vi "[FGV] Control_Eanble_Disable.vi"(7 "Control_EnDisable_Action":T2, 8 "Error In":errorcluster, 10 "Tab":T1=enum."Lookup Table", 11 "This VI":refnum<vi>) -> (0 "Error Out":errorcluster, 3 "PageRefOut":refnum<vi>)   [LabVIEW 2019]
uses:
  Controls/Control_EnDisable_Action.ctl
  Controls/UI_Process_Type.ctl
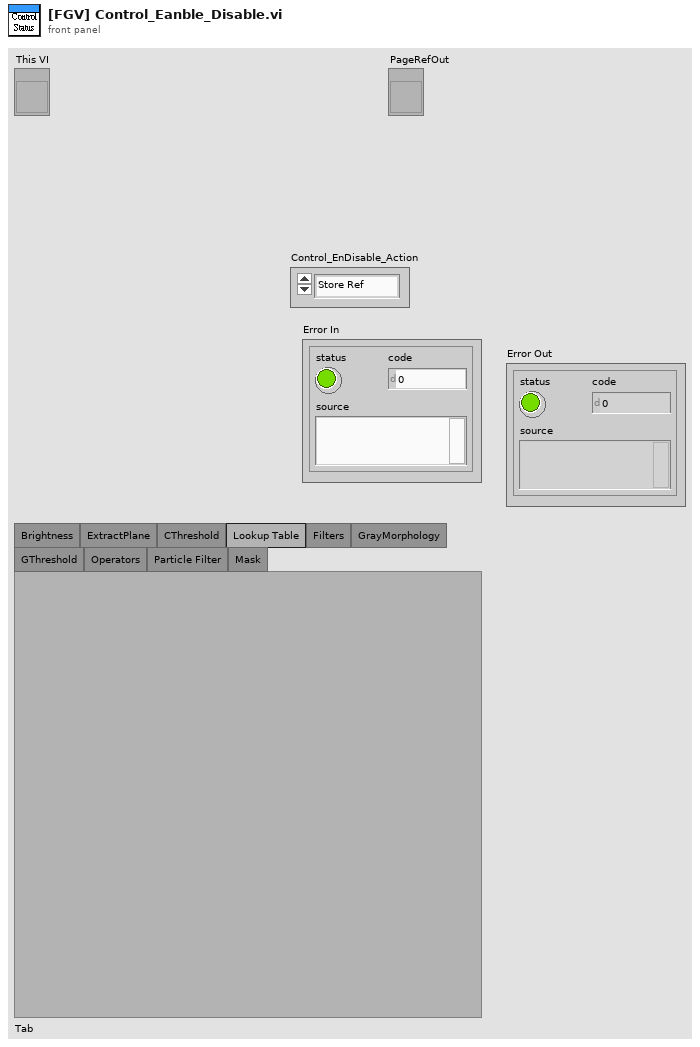
[diagram p1: front panel]
types:
  T1 = typedef "UI_Process_Type.ctl" = enum32{"None", "Brightness", "ExtractPlane", "CThreshold", "Lookup Table", "Filters", "GrayMorphology", "GThreshold", "Operators", "Particle Filter", "Mask"}
  T2 = typedef "Control_EnDisable_Action.ctl" = enum16{"Store Ref", "Add Mode", "Select Mode", "Enable All", "OnePageEnable", "OnePageDisable", "AllPageDisable", "AllPageEnable", "PageRefOut"}
  T3 = enum8{"Enabled", "Disabled", "Disabled and Grayed Out"}
  T4 = enum32{"Page Enabled", "Page Disabled", "Page Disabled & Grayed"}
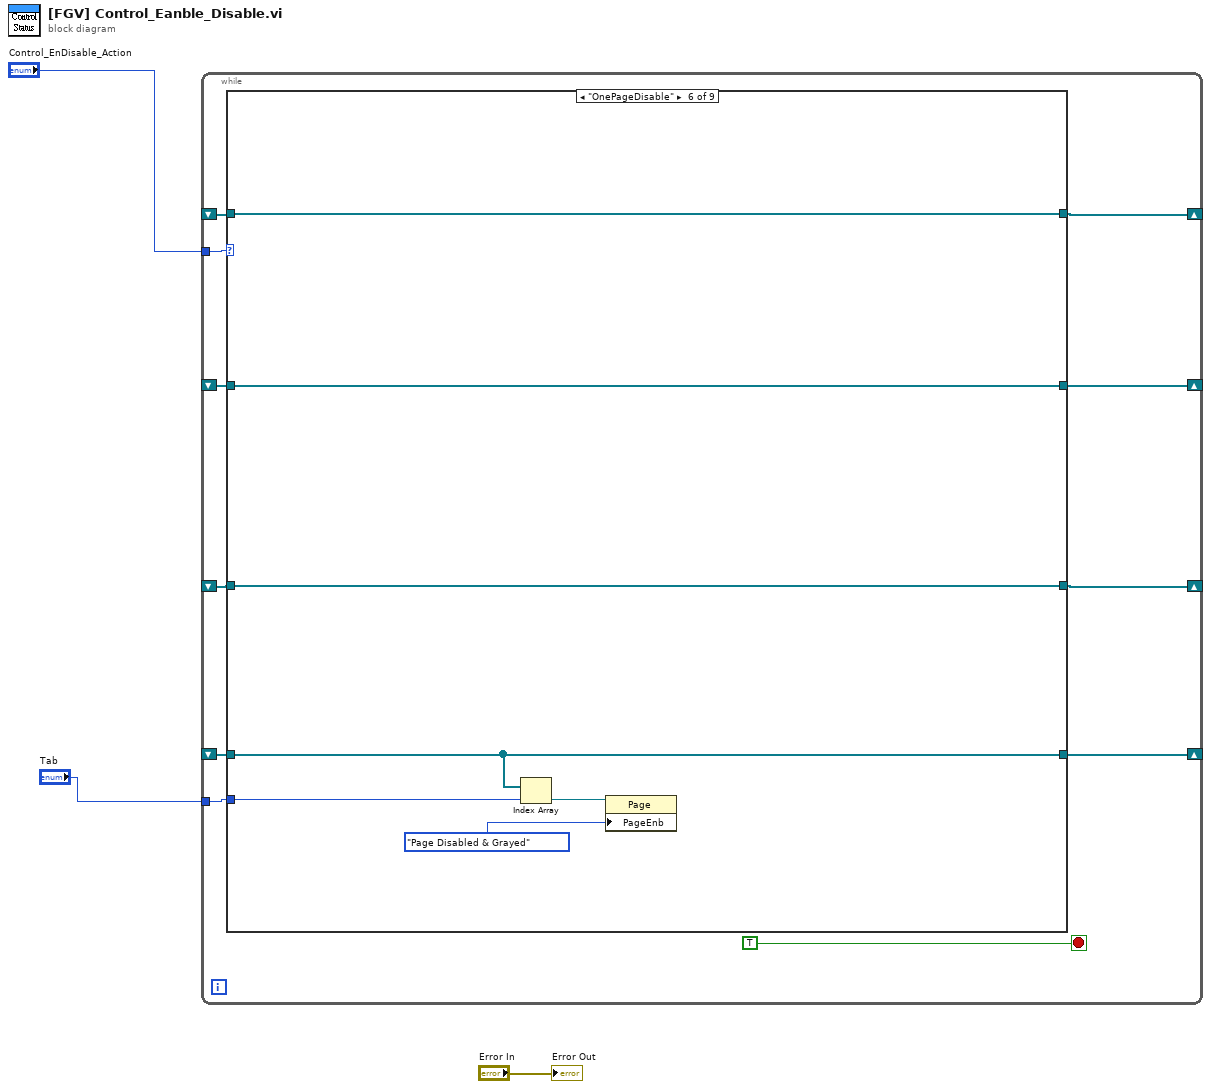
[diagram p0: block diagram]
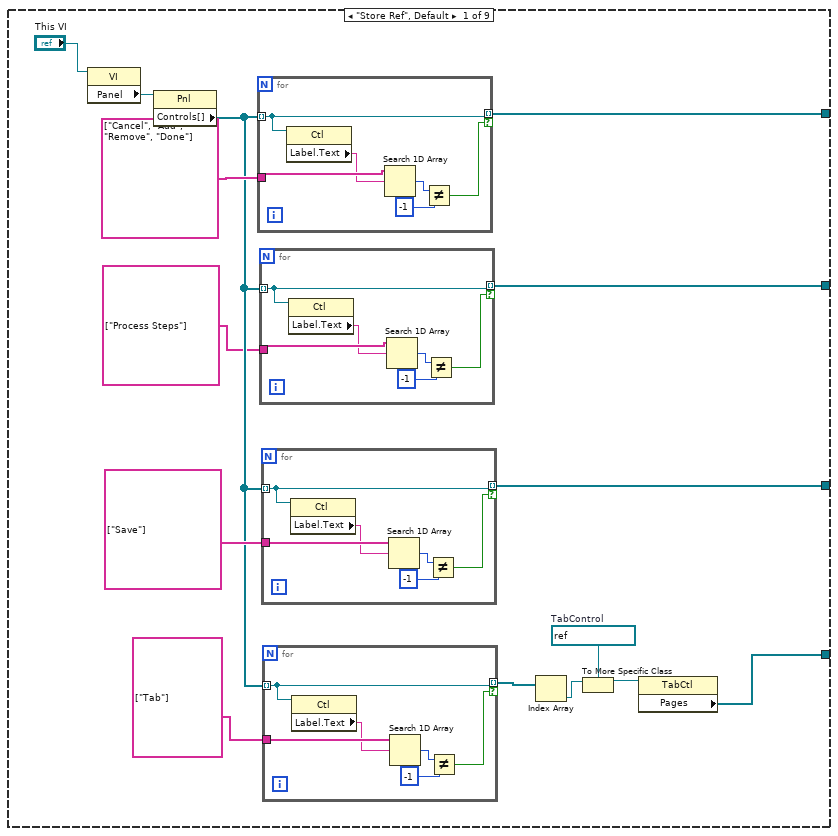
[diagram p2: hidden frame]
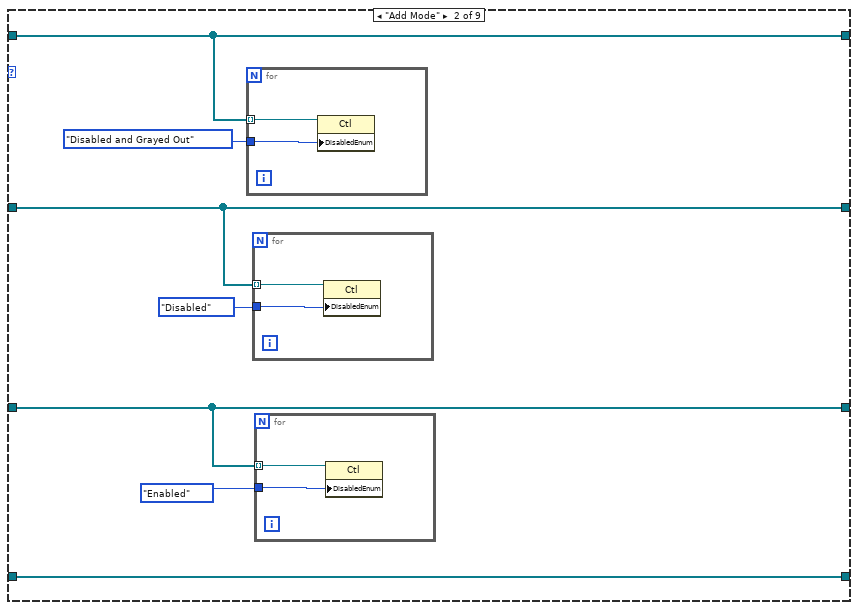
[diagram p3: hidden frame]
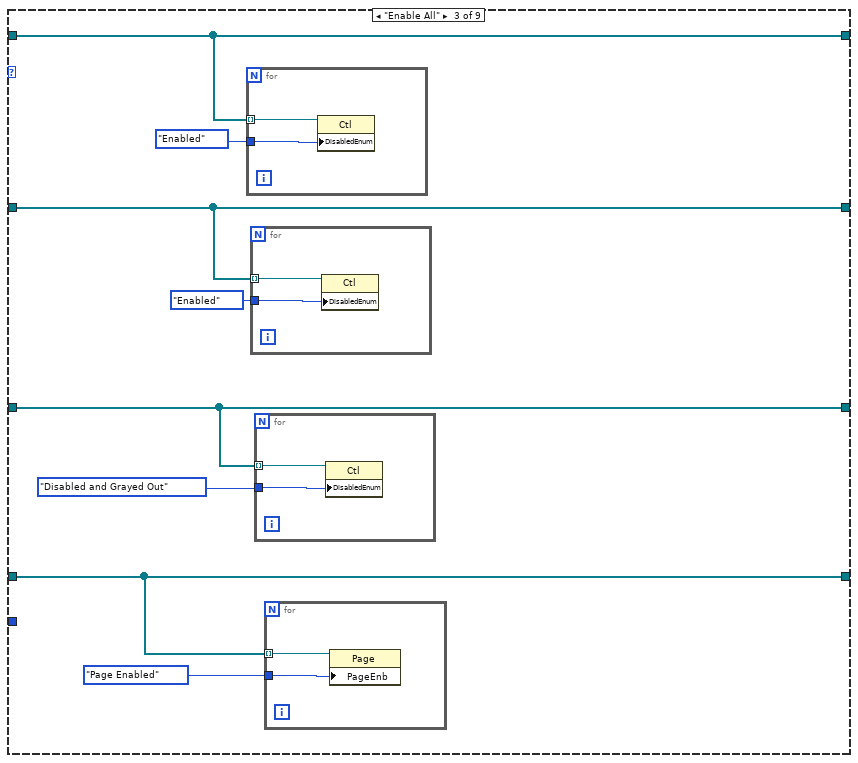
[diagram p4: hidden frame]
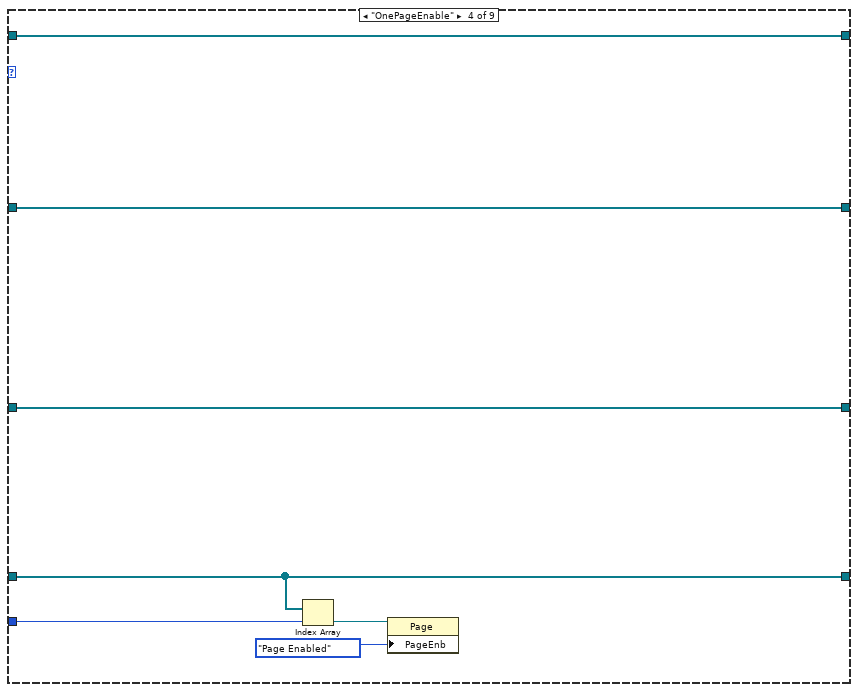
[diagram p5: hidden frame]
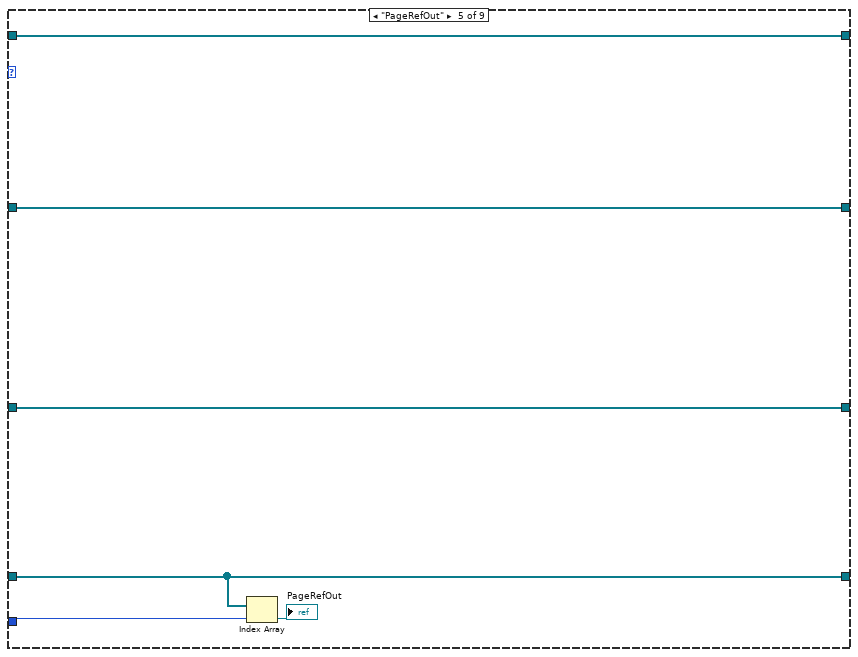
[diagram p6: hidden frame]
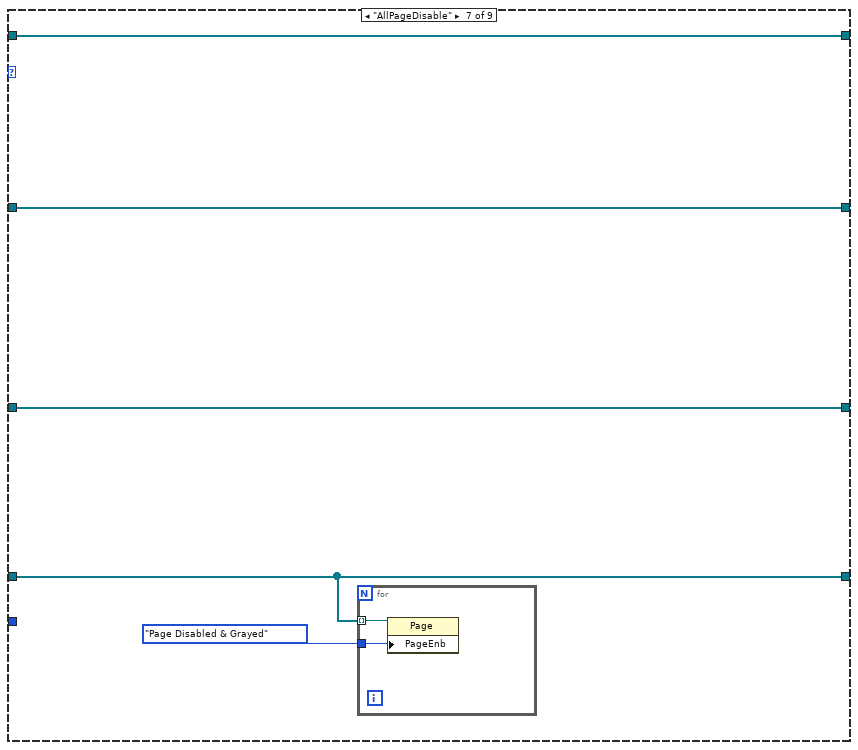
[diagram p7: hidden frame]
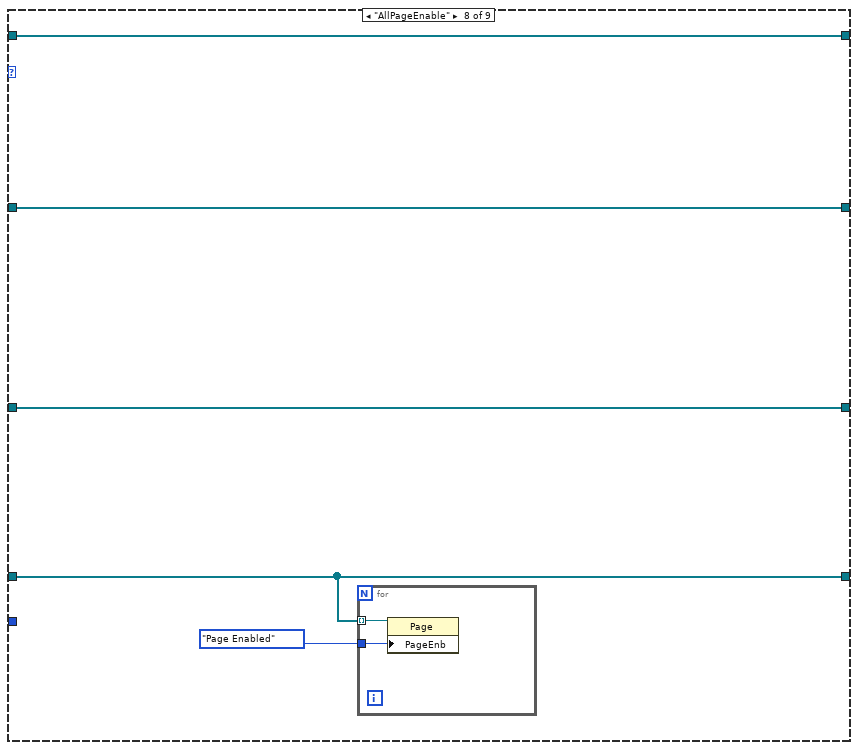
[diagram p8: hidden frame]
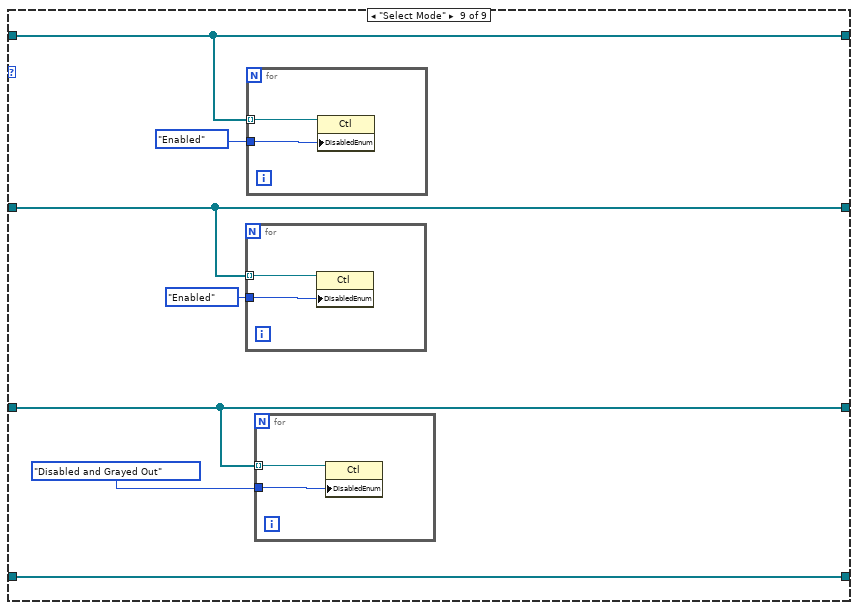
[diagram p9: hidden frame]
diagram:
  n1 = while {
    tunnel: "Control_EnDisable_Action" -> [w13]
    shift-right: [w12] -> _
    shift-left: _ -> [w9]
    shift-right: [w11] -> _
    shift-left: _ -> [w10]
    shift-right: [w8] -> _
    shift-left: _ -> [w7]
    tunnel: "Tab" -> [w6]
    shift-right: [w5] -> _
    shift-left: _ -> [w4]
    stop <- TRUE ("stop") stop-if-true
    n2 = case shown="\"OnePageDisable\"" w13 {
      tunnel: [w27 w58 w72 w89 w95 w102 w107 w114 w121] -> w12
      tunnel: w9 -> [_ w58 w72 w89 w95 w102 w107 w114 w121]
      tunnel: [w25 w57 w71 w88 w94 w101 w106 w113 w120] -> w11
      tunnel: w10 -> [_ w57 w71 w88 w94 w101 w106 w113 w120]
      tunnel: [w18 w56 w70 w87 w93 w100 w104 w111 w119] -> w8
      tunnel: w7 -> [_ w56 w70 w87 w93 w100 w104 w111 w119]
      tunnel: w6 -> [_ _ _ w84 w92 w97 _ _ _]
      tunnel: [w17 w55 w68 w83 w90 w96 w103 w110 w118] -> w5
      tunnel: w4 -> [_ w55 w68 w83 w90 w96 w103 w110 w118]
      frame "Store Ref", Default {
        w19 = refnum<vi> refnum  # TabControl
        n3 = property class="VI"(reference="This VI") -> ("Panel"=w29:refnum<vi>)  [unwired: 1 in, 2 out]
        n4 = property class="Pnl"(reference=w29) -> ("Controls[]"=w16:refnum<vi>[])  [unwired: 1 in, 2 out]
        n5 = for {
          tunnel: w16 -> [w49] mode=indexing
          tunnel: string[] ["Cancel", "Add", "Remove", "Done"] -> [w53]
          tunnel: [w49] -> w27 mode=indexing if=w48
          n6 = property class="Ctl"(reference=w49) -> ("Label.Text"=w50:string)  [unwired: 1 in, 2 out]
          n7 = Search 1D Array(1D array=w53, element=w50) -> (index of element=w52:i32)  [unwired: 1 in]
          n8 = Not Equal?(x=w52, y=-1) -> (x != y?=w48:bool)
        }
        n9 = for {
          tunnel: w16 -> [w31] mode=indexing
          tunnel: string[] ["Process Steps"] -> [w35]
          tunnel: [w31] -> w17 mode=indexing if=w30
          n10 = property class="Ctl"(reference=w31) -> ("Label.Text"=w32:string)  [unwired: 1 in, 2 out]
          n11 = Search 1D Array(1D array=w35, element=w32) -> (index of element=w34:i32)  [unwired: 1 in]
          n12 = Not Equal?(x=w34, y=-1) -> (x != y?=w30:bool)
        }
        n13 = for {
          tunnel: w16 -> [w43] mode=indexing
          tunnel: string[] ["Save"] -> [w47]
          tunnel: [w43] -> w25 mode=indexing if=w42
          n14 = property class="Ctl"(reference=w43) -> ("Label.Text"=w44:string)  [unwired: 1 in, 2 out]
          n15 = Search 1D Array(1D array=w47, element=w44) -> (index of element=w46:i32)  [unwired: 1 in]
          n16 = Not Equal?(x=w46, y=-1) -> (x != y?=w42:bool)
        }
        n17 = for {
          tunnel: w16 -> [w37] mode=indexing
          tunnel: string[] ["Tab"] -> [w41]
          tunnel: [w37] -> w22 mode=indexing if=w36
          n18 = property class="Ctl"(reference=w37) -> ("Label.Text"=w38:string)  [unwired: 1 in, 2 out]
          n19 = Search 1D Array(1D array=w41, element=w38) -> (index of element=w40:i32)  [unwired: 1 in]
          n20 = Not Equal?(x=w40, y=-1) -> (x != y?=w36:bool)
        }
        n21 = Index Array(array=w22) -> (element=w21:refnum<vi>)  [unwired: 1 in]
        n22 = To More Specific Class(target class=w19, reference=w21) -> (specific class reference=w20:refnum<vi>)  [unwired: 1 in, 1 out]
        n23 = property class="TabCtl"(reference=w20) -> ("Pages"=w18:refnum<vi>[])  [unwired: 1 in, 2 out]
      }
      frame "Add Mode" {
        n24 = for {
          tunnel: w58 -> [w66] mode=indexing
          tunnel: T3."Disabled and Grayed Out" ("Disabled") -> [w65]
          n25 = property class="Ctl"(reference=w66, "DisabledEnum"=w65) -> ()  [unwired: 1 in, 2 out]
        }
        n26 = for {
          tunnel: w55 -> [w62] mode=indexing
          tunnel: T3."Disabled" ("Disabled") -> [w61]
          n27 = property class="Ctl"(reference=w62, "DisabledEnum"=w61) -> ()  [unwired: 1 in, 2 out]
        }
        n28 = for {
          tunnel: w57 -> [w64] mode=indexing
          tunnel: T3."Enabled" ("Disabled") -> [w63]
          n29 = property class="Ctl"(reference=w64, "DisabledEnum"=w63) -> ()  [unwired: 1 in, 2 out]
        }
      }
      frame "Enable All" {
        n30 = for {
          tunnel: w72 -> [w82] mode=indexing
          tunnel: T3."Enabled" ("Disabled") -> [w81]
          n31 = property class="Ctl"(reference=w82, "DisabledEnum"=w81) -> ()  [unwired: 1 in, 2 out]
        }
        n32 = for {
          tunnel: w68 -> [w76] mode=indexing
          tunnel: T3."Enabled" ("Disabled") -> [w75]
          n33 = property class="Ctl"(reference=w76, "DisabledEnum"=w75) -> ()  [unwired: 1 in, 2 out]
        }
        n34 = for {
          tunnel: w71 -> [w80] mode=indexing
          tunnel: T3."Disabled and Grayed Out" ("Disabled") -> [w79]
          n35 = property class="Ctl"(reference=w80, "DisabledEnum"=w79) -> ()  [unwired: 1 in, 2 out]
        }
        n36 = for {
          tunnel: w70 -> [w78] mode=indexing
          tunnel: T4."Page Enabled" ("Page Enabled State") -> [w77]
          n37 = property class="Page"(reference=w78, "PageEnb"=w77) -> ()  [unwired: 1 in, 2 out]
        }
      }
      frame "OnePageEnable" {
        n38 = Index Array(array=w87, index=w84) -> (element=w86:refnum<vi>)
        n39 = property class="Page"(reference=w86, "PageEnb"=T4."Page Enabled" ("Page Enabled State")) -> ()  [unwired: 1 in, 2 out]
      }
      frame "PageRefOut" {
        n40 = Index Array(array=w93, index=w92) -> (element=→"PageRefOut":refnum<vi>)
      }
      frame "OnePageDisable" {
        n41 = Index Array(array=w100, index=w97) -> (element=w99:refnum<vi>)
        n42 = property class="Page"(reference=w99, "PageEnb"=T4."Page Disabled & Grayed" ("Page Enabled State")) -> ()  [unwired: 1 in, 2 out]
      }
      frame "AllPageDisable" {
        n43 = for {
          tunnel: T4."Page Disabled & Grayed" ("Page Enabled State") -> [w109]
          tunnel: w104 -> [w108] mode=indexing
          n44 = property class="Page"(reference=w108, "PageEnb"=w109) -> ()  [unwired: 1 in, 2 out]
        }
      }
      frame "AllPageEnable" {
        n45 = for {
          tunnel: T4."Page Enabled" ("Page Enabled State") -> [w116]
          tunnel: w111 -> [w115] mode=indexing
          n46 = property class="Page"(reference=w115, "PageEnb"=w116) -> ()  [unwired: 1 in, 2 out]
        }
      }
      frame "Select Mode" {
        n47 = for {
          tunnel: w118 -> [w125] mode=indexing
          tunnel: T3."Enabled" ("Disabled") -> [w124]
          n48 = property class="Ctl"(reference=w125, "DisabledEnum"=w124) -> ()  [unwired: 1 in, 2 out]
        }
        n49 = for {
          tunnel: w121 -> [w129] mode=indexing
          tunnel: T3."Enabled" ("Disabled") -> [w128]
          n50 = property class="Ctl"(reference=w129, "DisabledEnum"=w128) -> ()  [unwired: 1 in, 2 out]
        }
        n51 = for {
          tunnel: w120 -> [w127] mode=indexing
          tunnel: T3."Disabled and Grayed Out" ("Disabled") -> [w126]
          n52 = property class="Ctl"(reference=w127, "DisabledEnum"=w126) -> ()  [unwired: 1 in, 2 out]
        }
      }
    }
  }
  "Error Out" <- "Error In"
